vi "get #OfNorms.vi"(8 "error in (no error)":errorcluster caption="Fehler (Eingang, kein Fehler)", 11 "Report (Eingang)":refnum<class "Report.lvclass">) -> (0 "error out":errorcluster caption="Fehler (Ausgang)", 2 "#OfTests":u32, 3 "Report (Ausgang)":refnum<class "Report.lvclass">)   [LabVIEW 2013, in "DatenKlassen.lvlib" / "Report.lvclass"]
uses:
  Report.lvclass
  Report.lvclass/Report.ctl
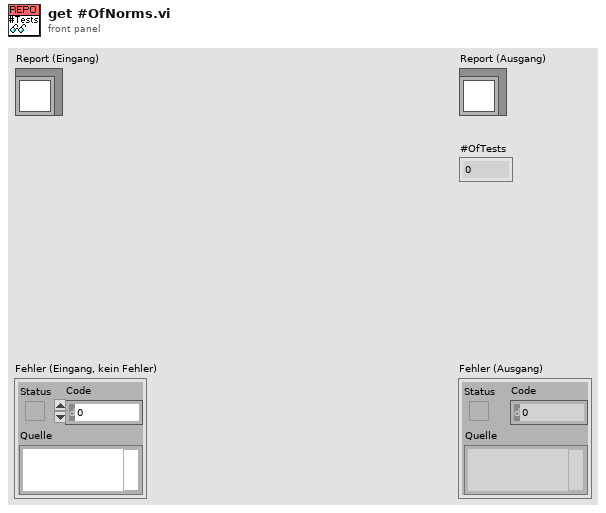
[diagram p1: front panel]
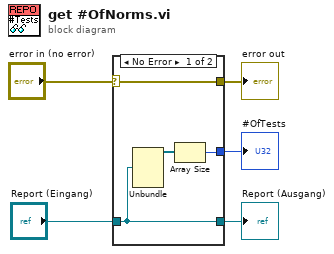
[diagram p0: block diagram]
diagram:
  n1 = case shown="No Error" "error in (no error)" {
    selector: "error in (no error)" -> [w9 w10]
    tunnel: [w9 w10] -> w4
    tunnel: [w8 w11] -> w2
    tunnel: "Report (Eingang)" -> [w8 w11]
    tunnel: [w7 _] -> w1
    frame No Error {
      n2 = Unbundle(w8) -> (w6:refnum<class "Norm.lvclass">[])  [unwired: 4 out]
      n3 = Array Size(array=w6) -> (size(s)=w7:i32)
    }
    frame Error {
    }
  }
  "error out" <- w4
  "Report (Ausgang)" <- w2
  "#OfTests" <- w1
